vi "PerfResize.vi"() -> ()   [LabVIEW 2024, in "TypedCircularBuffer.Tests.Perf.lvlib"]
uses:
  TypedCircularBuffer.Tests.Perf.lvlib
  <vilib>/Analysis/NI_AALBase.lvlib
  TypedCircularBuffer.lvclass
  <vilib>/Analysis/baseanly.llb/Mean (DBL).vi
panel:
  out "resize time":dbl format="%.2p"
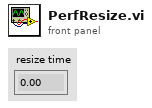
[diagram p1: front panel]
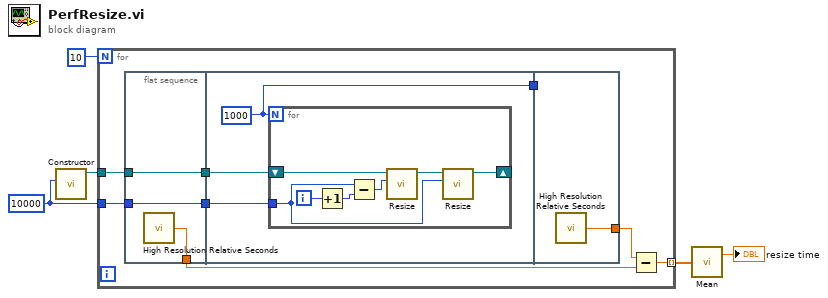
[diagram p0: block diagram]
diagram:
  w1 = u32 10000 ("Capacity")
  n1 = call "Constructor.vi"("Capacity"=w1) -> ("TypedCircularBuffer out"=w4:refnum<class "TypedCircularBuffer.lvclass">)  [unwired: 10 in]
  n2 = for {
    N: 10 -> [_]
    tunnel: w4 -> [w13]
    tunnel: [w8] -> w2 mode=indexing
    tunnel: w1 -> [w7]
    n3 = flat-sequence {
      tunnel: w13 -> [w16]
      tunnel: [w16] -> w11
      tunnel: [w15] -> w9
      tunnel: w7 -> [w14]
      tunnel: [w14] -> w6
      tunnel: [w18] -> w12
      tunnel: w11 -> [w19]
      tunnel: w6 -> [w17]
      tunnel: w12 -> [_]
      tunnel: [w27] -> w10
      frame #0 {
        n4 = call <vilib>:"High Resolution Relative Seconds.vi"() -> ("relative seconds"=w15:dbl)
      }
      frame #1 {
        w18 = 1000
        n5 = for {
          N: w18 -> [_]
          shift-right: [w21] -> _
          shift-left: w19 -> [w26]
          tunnel: w17 -> [w20]
          i -> [w25]
          n6 = Increment(x=w25) -> (x+1=w23:i32)
          n7 = Subtract(x=w20, y=w23) -> (x-y=w24:u32)
          n8 = call "Resize.vi"("Capacity"=w24, "TypedCircularBuffer in"=w26) -> ("TypedCircularBuffer out"=w22:refnum<class "TypedCircularBuffer.lvclass">)  [unwired: 9 in]
          n9 = call "Resize.vi"("Capacity"=w20, "TypedCircularBuffer in"=w22) -> ("TypedCircularBuffer out"=w21:refnum<class "TypedCircularBuffer.lvclass">)  [unwired: 9 in]
        }
      }
      frame #2 {
        n10 = call <vilib>:"High Resolution Relative Seconds.vi"() -> ("relative seconds"=w27:dbl)
      }
    }
    n11 = Subtract(x=w10, y=w9) -> (x-y=w8:dbl)
  }
  n12 = call-poly <vilib>:"Mean.vi"("X"=w2) -> ("mean"=→"resize time":dbl)  [unwired: 1 out]
